vi "Init Data Object.vi"(11 "CRDS Cell Data in":refnum<class "CRDS Cell Data.lvclass">) -> (3 "CRDS Cell Data out":refnum<class "CRDS Cell Data.lvclass">)   [LabVIEW 2014, in "CRDS Cell Data.lvclass"]
uses:
  CRDS Cell Data.lvclass
  Data/Data.lvclass/Data.ctl
  CRDS Cell Data.lvclass/CRDS Cell Data.ctl
  Data/Data.lvclass
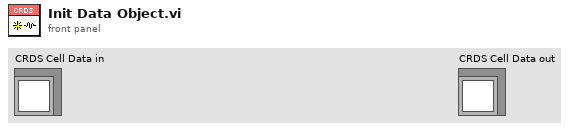
[diagram p1: front panel]
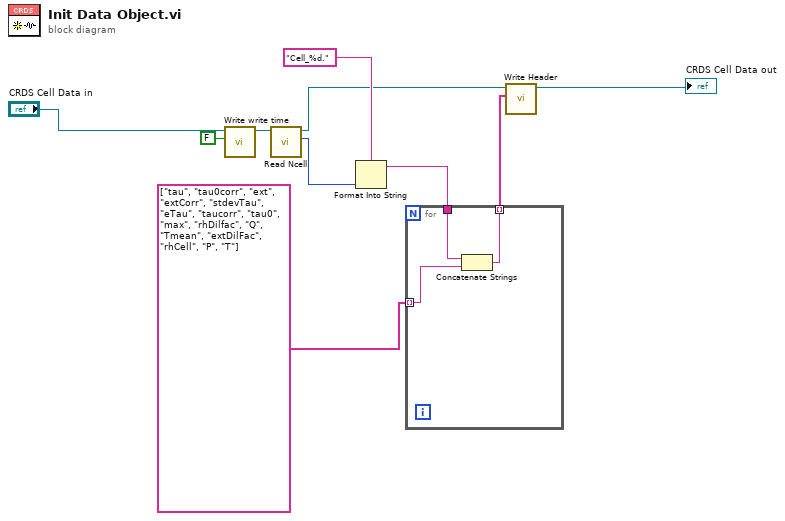
[diagram p0: block diagram]
diagram:
  n1 = call "Write write time.vi"("write time"=FALSE, "Data in"="CRDS Cell Data in") -> ("Data out"=w8:refnum<class "CRDS Cell Data.lvclass">)  [unwired: 8 in, 1 out]
  n2 = call "Read Ncell.vi"("CRDS Cell Data in"=w8) -> ("Ncell"=w6:u8, "CRDS Cell Data out"=w2:refnum<class "CRDS Cell Data.lvclass">)  [unwired: 8 in, 1 out]
  n3 = Format Into String(format string="Cell_%d.", w6) -> (resulting string=w4:string)  [unwired: 2 in, 1 out]
  n4 = for {
    tunnel: string[] ["tau", "tau0corr", "ext", "extCorr", "stdevTau", "eTau", "taucorr", "tau0", "max", "rhDilfac", "Q", "Tmean", "extDilFac", "rhCell", "P", "T"] -> [w12] mode=indexing
    tunnel: w4 -> [w13]
    tunnel: [w11] -> w3 mode=indexing
    n5 = Concatenate Strings(w13, w12) -> (w11:string)
  }
  n6 = call "Write Header.vi"("Header"=w3, "Data in"=w2) -> ("Data out"=→"CRDS Cell Data out":refnum<class "CRDS Cell Data.lvclass">)  [unwired: 8 in, 1 out]
